vi "eval.vi"(8 "Environment in":T1, 9 "Expression in":T2) -> (2 "Environment out":T1, 3 "Expression out":T2)   [LabVIEW 2020]
uses:
  ExpressionType.ctl
  Expression.ctl
  ClosureData.ctl
  Environment.ctl
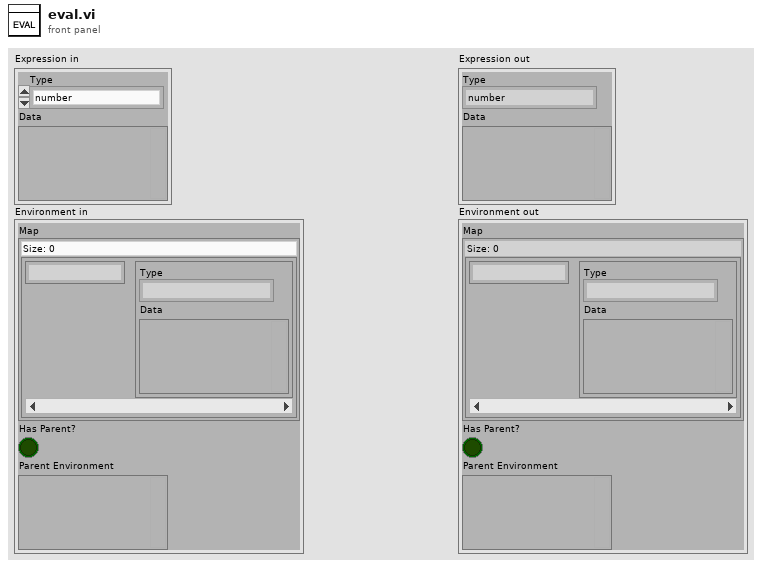
[diagram p1: front panel]
types:
  T1 = typedef "Environment.ctl" = cluster{"Map":map{string, T2}, "Has Parent?":bool, "Parent Environment":variant}
  T2 = typedef "Expression.ctl" = cluster{"Type":T3, "Data":variant}
  T3 = typedef "ExpressionType.ctl" = enum16{"number", "string", "symbol", "primitive", "list", "closure", "macro", "nil", "error"}
  T4 = typedef "ClosureData.ctl" = cluster{"arguments":string[], "code":T2}
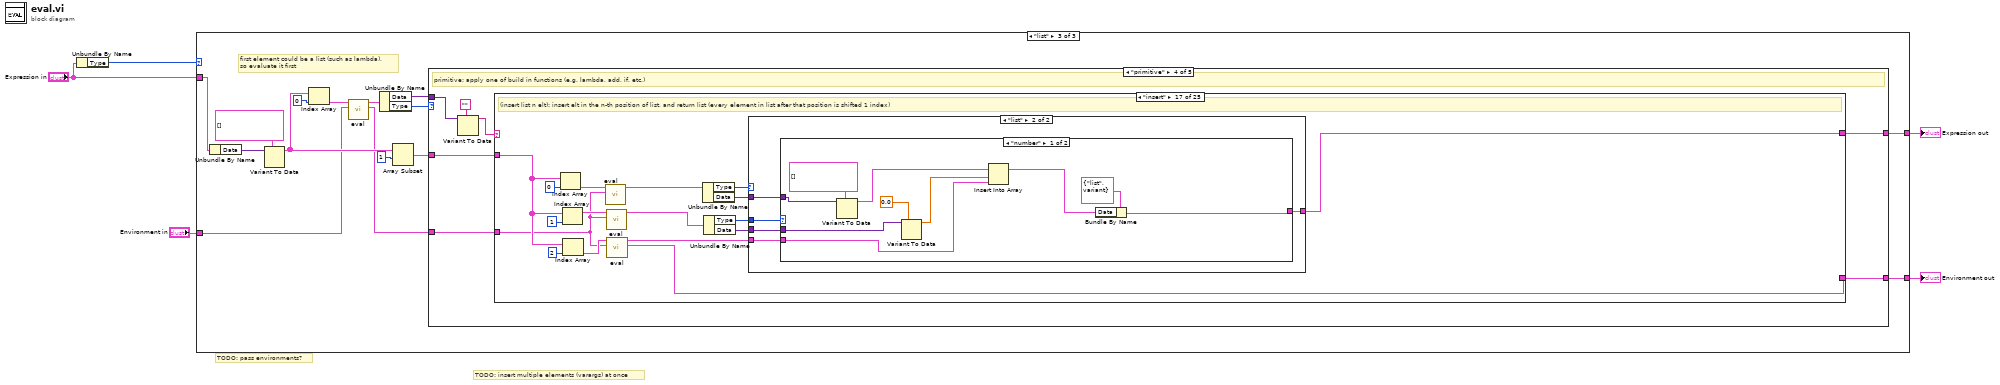
[diagram p0: block diagram]
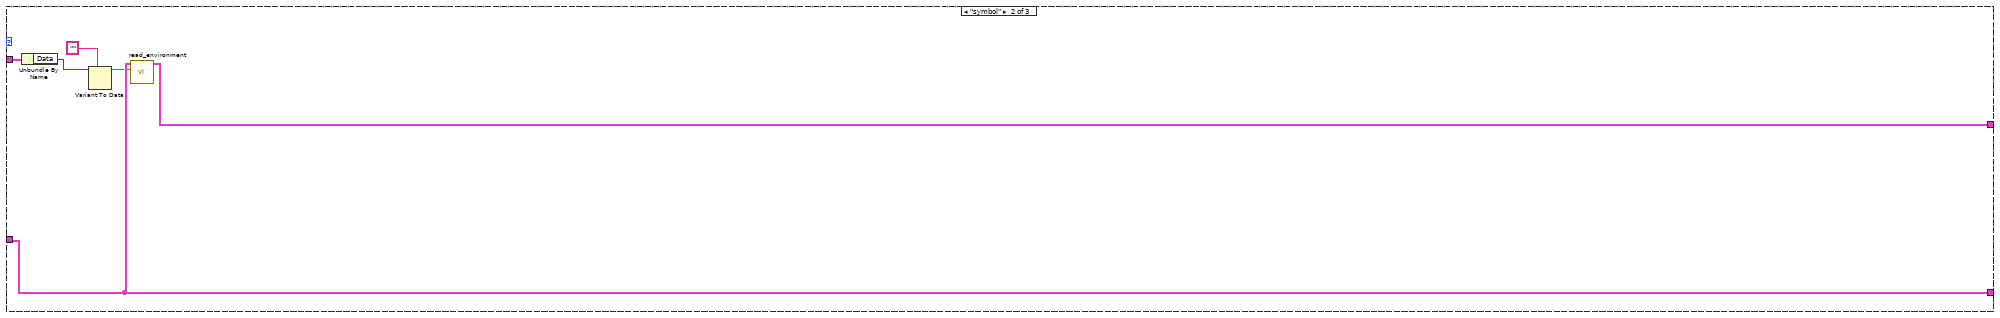
[diagram p3: hidden frame]
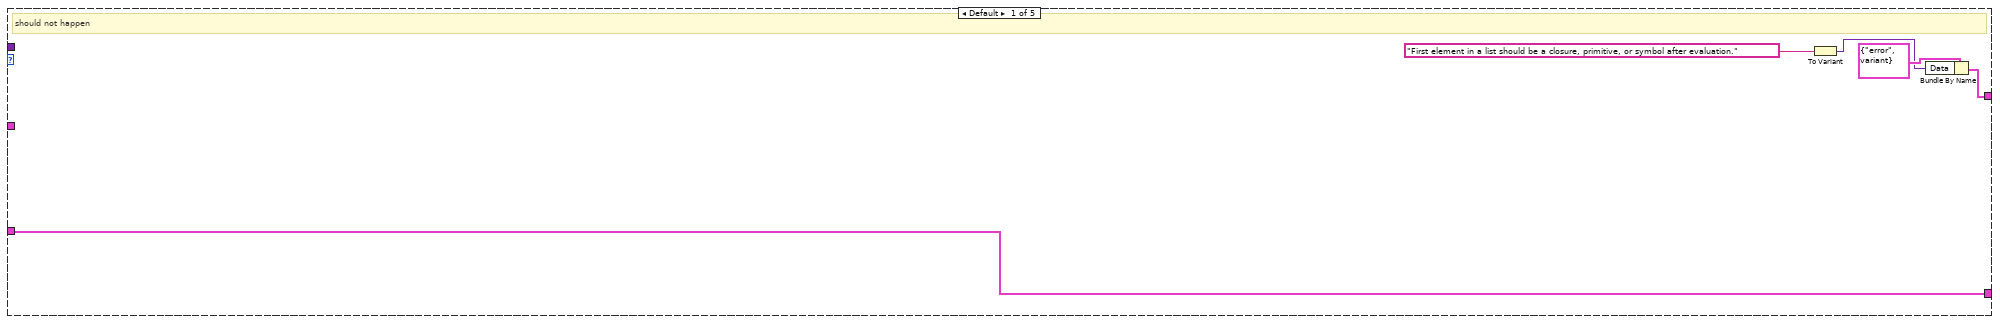
[diagram p4: hidden frame]
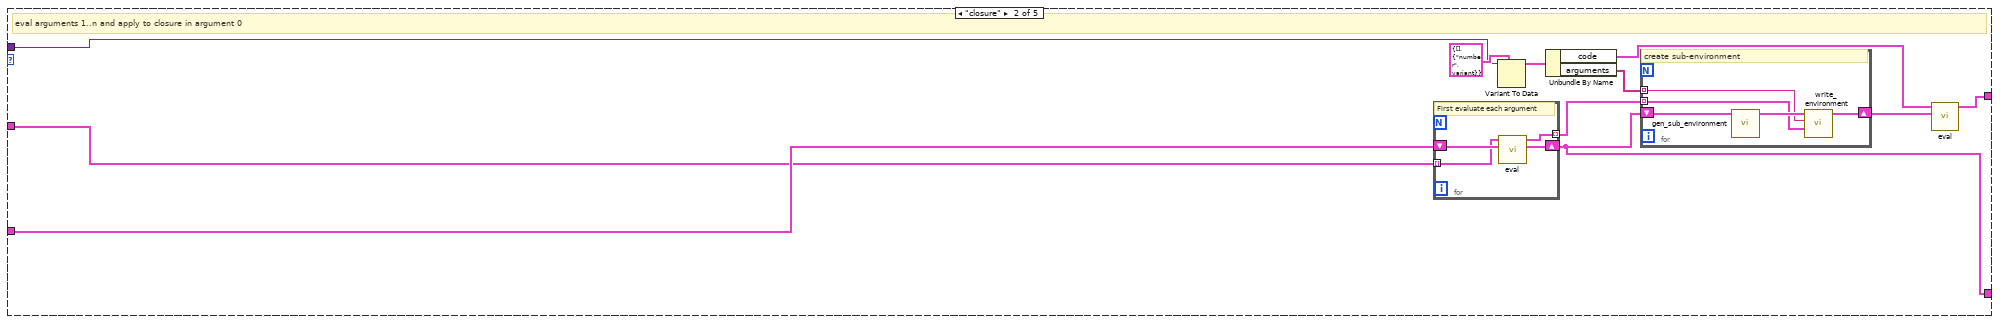
[diagram p5: hidden frame]
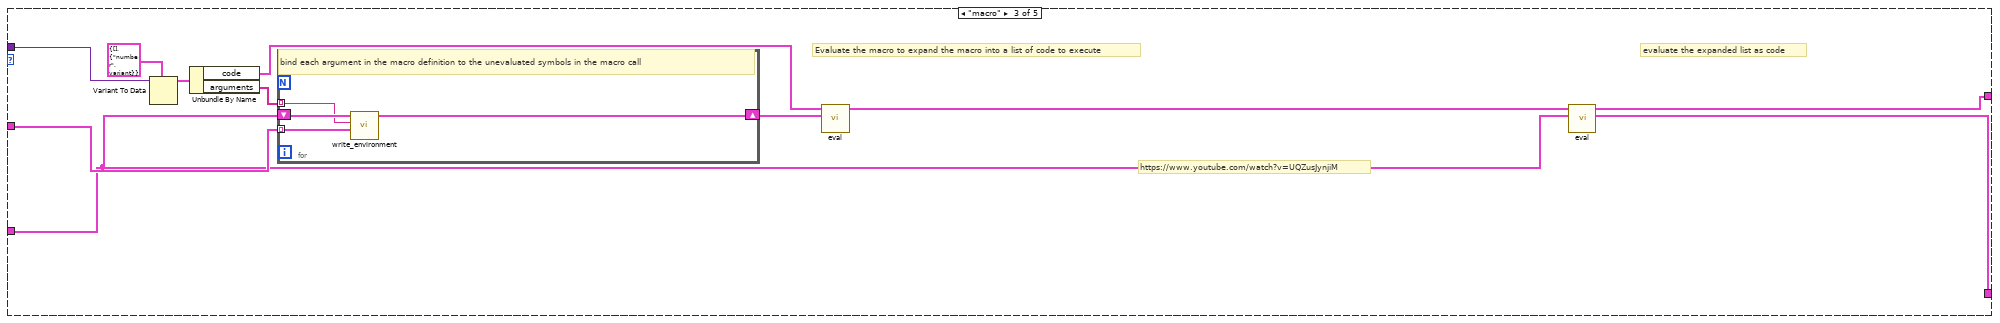
[diagram p6: hidden frame]
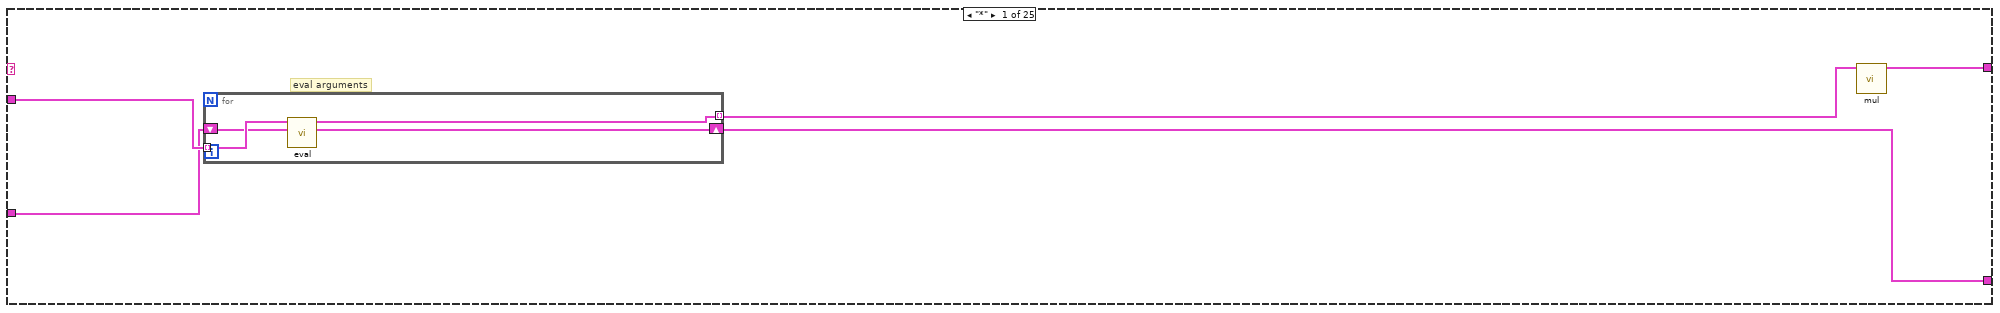
[diagram p7: hidden frame]
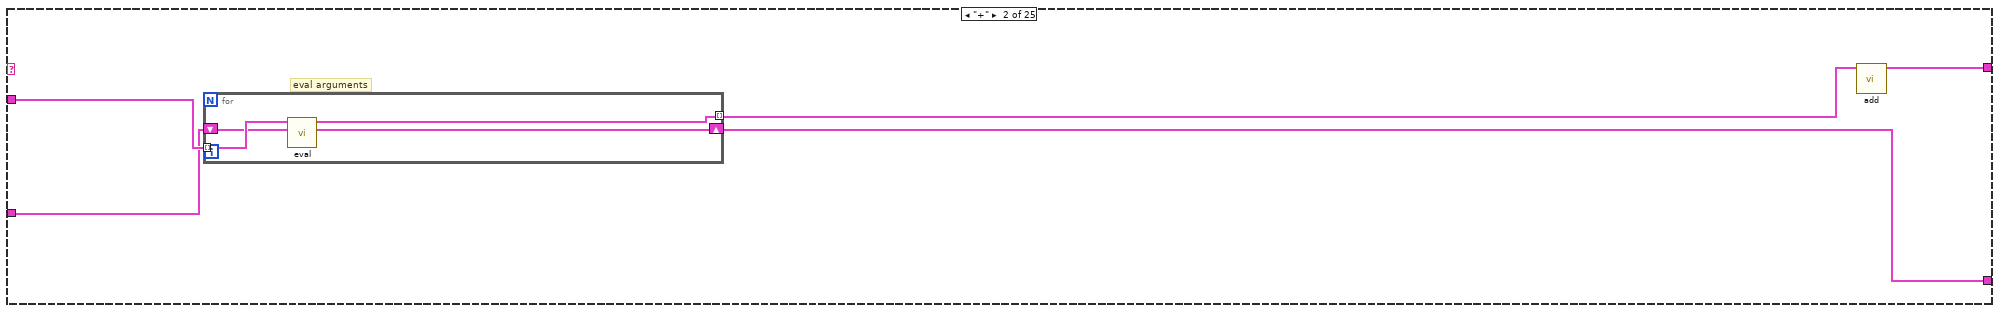
[diagram p8: hidden frame]
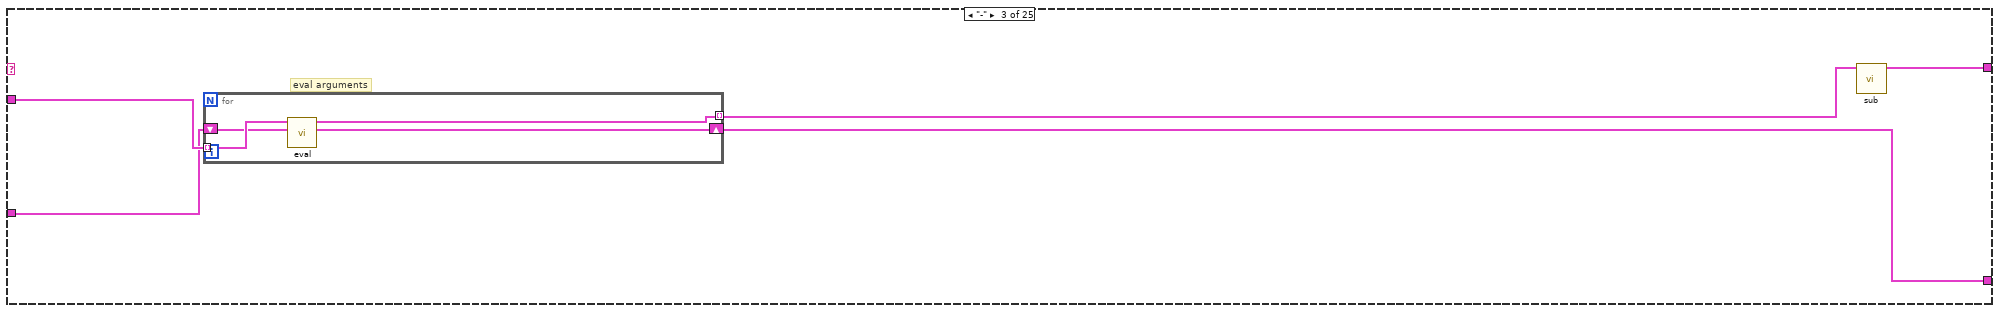
[diagram p9: hidden frame]
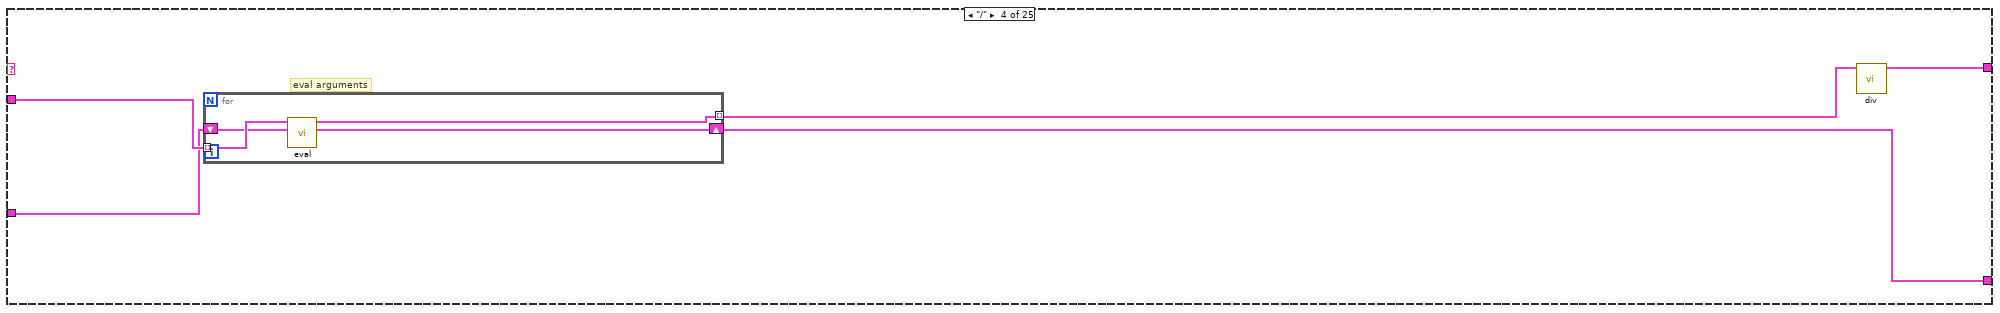
[diagram p10: hidden frame]
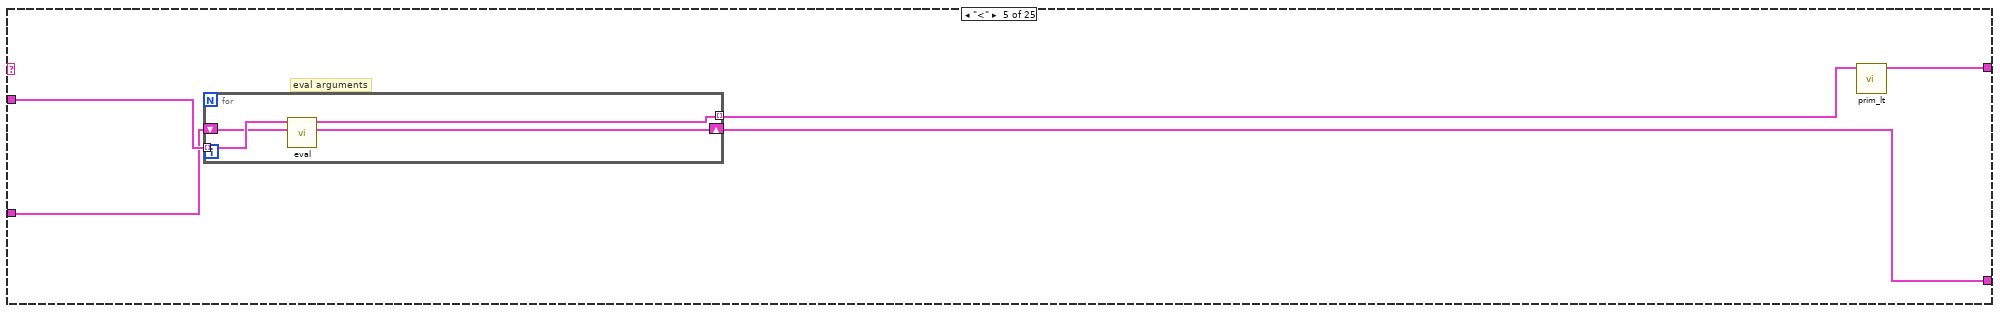
[diagram p11: hidden frame]
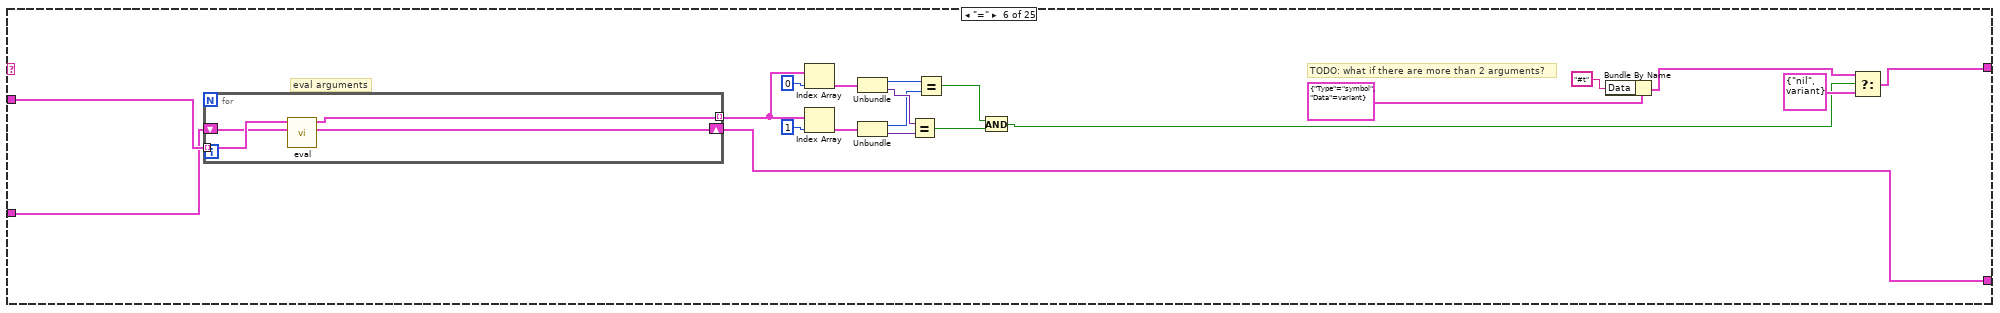
[diagram p12: hidden frame]
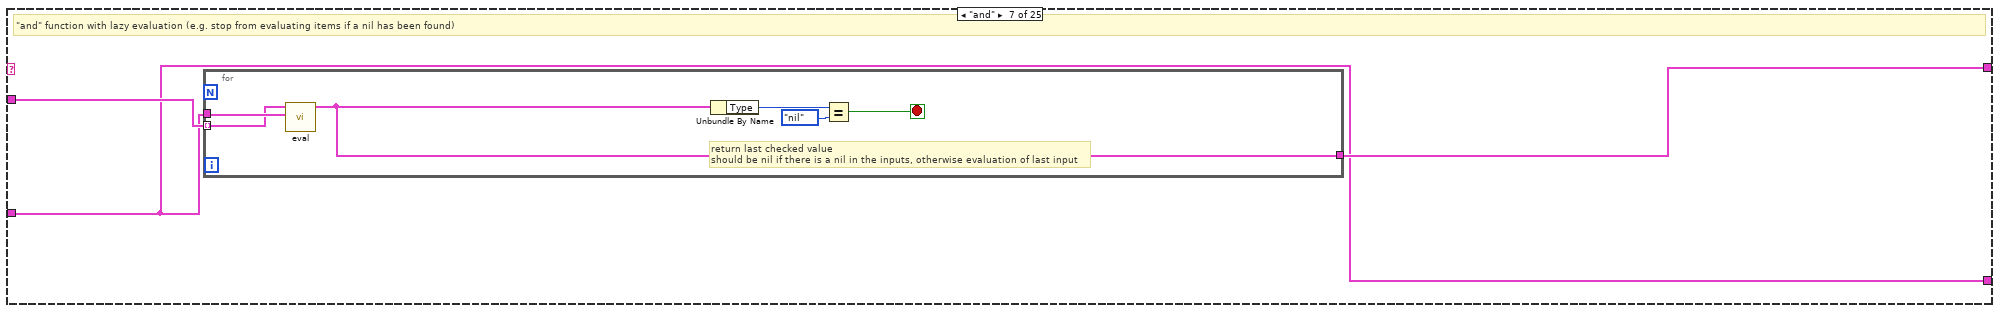
[diagram p13: hidden frame]
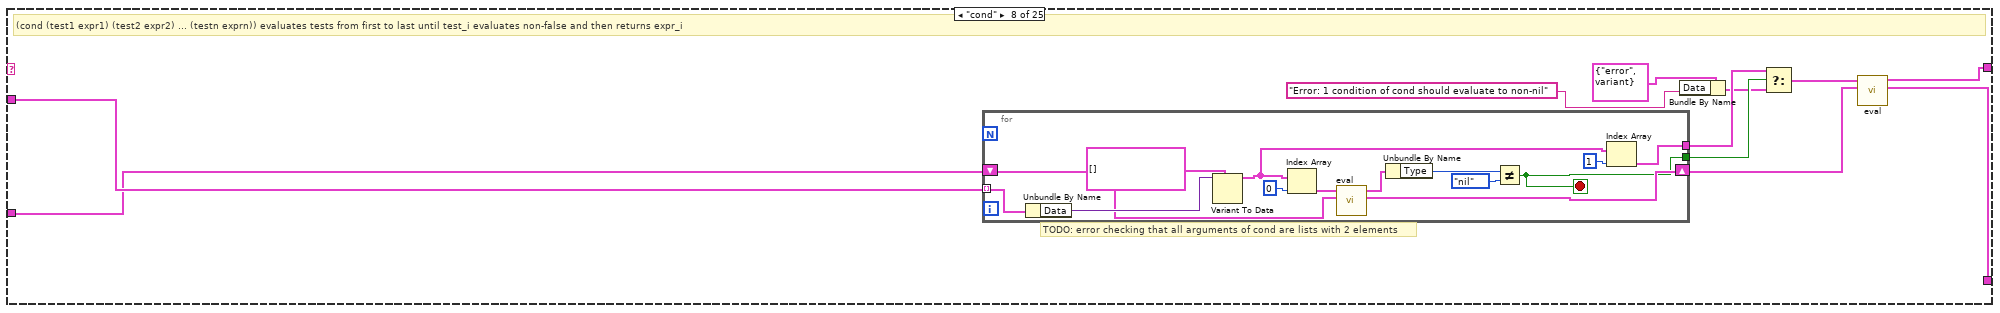
[diagram p14: hidden frame]
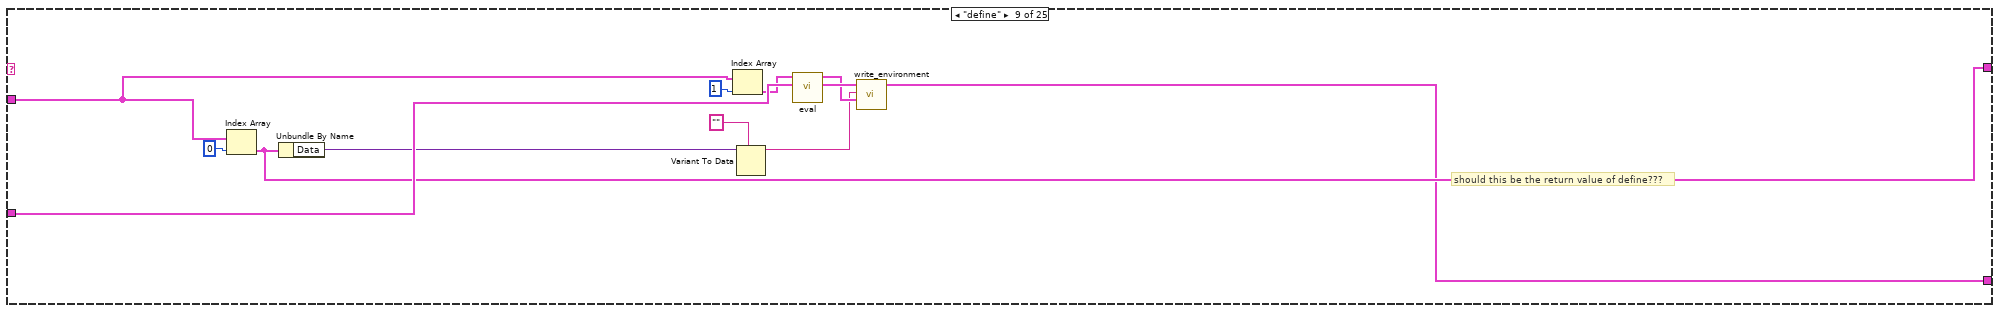
[diagram p15: hidden frame]
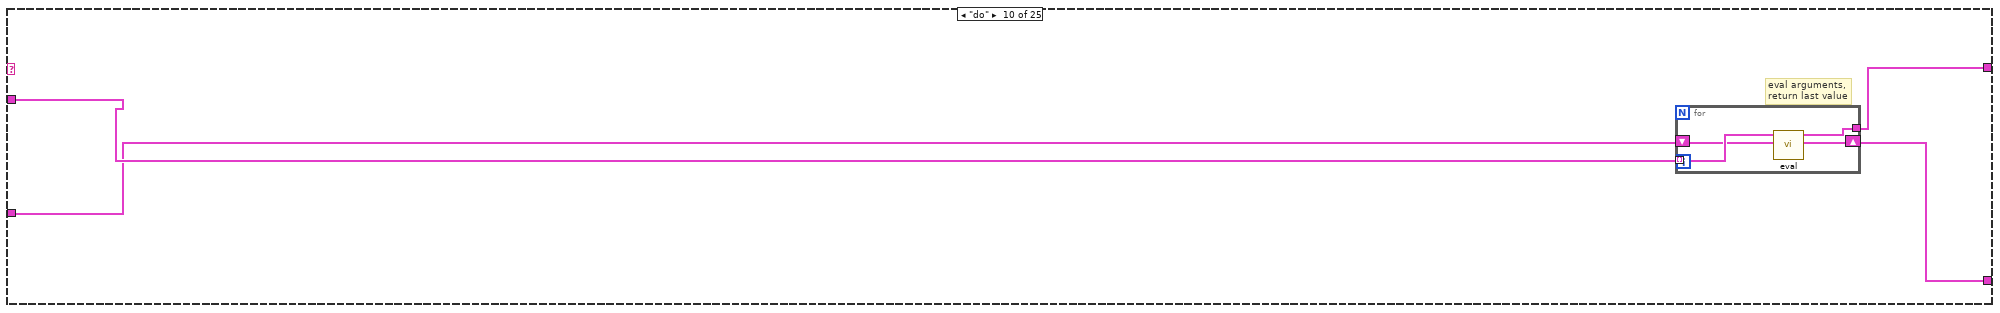
[diagram p16: hidden frame]
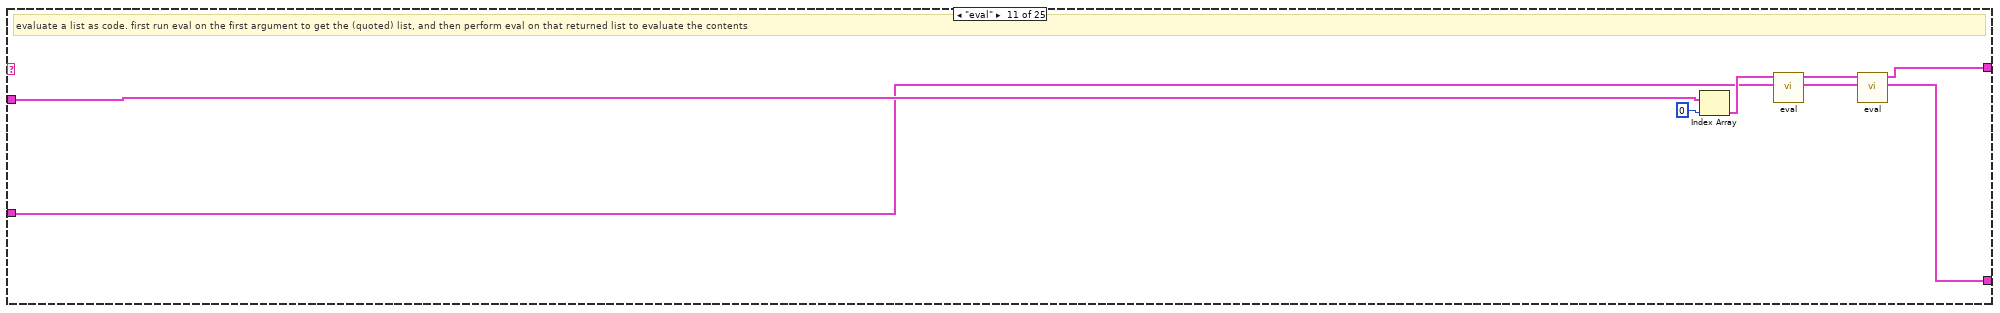
[diagram p17: hidden frame]
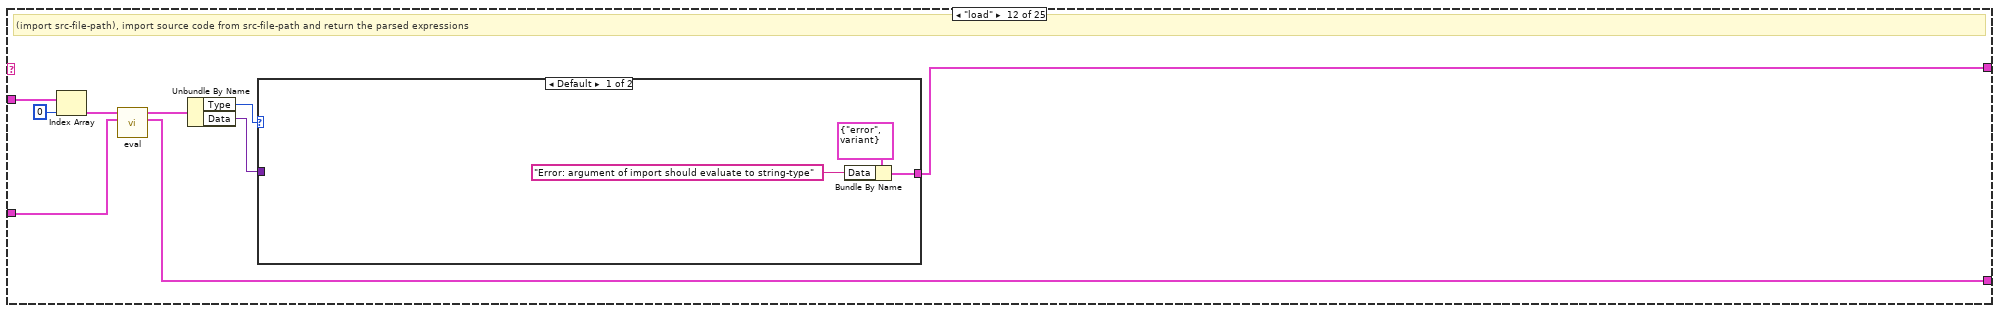
[diagram p18: hidden frame]
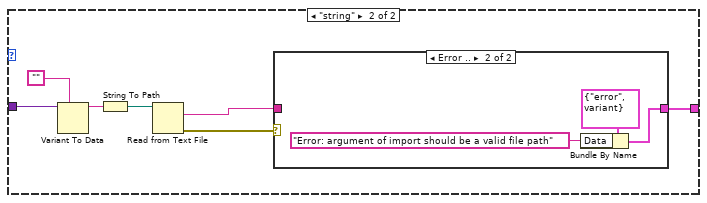
[diagram p19: hidden frame]
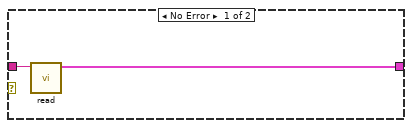
[diagram p20: hidden frame]
diagram:
  # "TODO: insert multiple elements (varargs) at once"
  # "TODO: pass environments?"
  n1 = Unbundle By Name("Expression in") -> ("Type"=w4:T3)
  n2 = case shown="\"list\"" w4 {
    tunnel: "Expression in" -> [w7 w9 w15]
    tunnel: [w7 w11 w25] -> w3
    tunnel: "Environment in" -> [w6 w12 w17]
    tunnel: [w6 w12 w16] -> w1
    frame "number", "string", "primitive", "closure".."error" {
    }
    frame "symbol" {
      n3 = Unbundle By Name(w9) -> ("Data"=w8:variant)
      n4 = Variant To Data(type="", Variant=w8) -> (data=w10:string)  [unwired: 1 in, 1 out]
      n5 = call "read_environment.vi"("symbol"=w10, "Environment in"=w12) -> ("Expression"=w11:T2)  [unwired: 9 in]
    }
    frame "list" {
      # "first element could be a list (such as lambda),\nso evaluate it first"
      n6 = Unbundle By Name(w15) -> ("Data"=w14:variant)
      n7 = Variant To Data(type=T2[] [], Variant=w14) -> (data=w23:T2[])  [unwired: 1 in, 1 out]
      n8 = Index Array(array=w23, index=0) -> (element=w19:T2)
      n9 = call "eval.vi"("Environment in"=w17, "Expression in"=w19) -> ("Environment out"=w20:T1, "Expression out"=w18:T2)  [unwired: 6 in]
      n10 = Unbundle By Name(w18) -> ("Data"=w26:variant, "Type"=w21:T3)
      n11 = Array Subset(array=w23, index=1) -> (w22:T2[])  [unwired: 1 in]
      n12 = case shown="\"primitive\"" w21 {
        tunnel: w26 -> [_ w41 w63 w74 w476]
        tunnel: w20 -> [w33 w44 w57 w70 w474]
        tunnel: [w29 w34 w54 w72 w472] -> w25
        tunnel: w22 -> [_ w43 w60 w71 _]
        tunnel: [w33 w37 w55 w69 w474] -> w16
        frame Default {
          # "should not happen"
          n13 = To Variant(anything="First element in a list should be a closure, primitive, or symbol after evaluation.") -> (Variant=w31:variant)
          n14 = Bundle By Name(cluster=T2 {"Type"=enum."error", "Data"=variant} ("Expression out"), "Data"=w31) -> (w29:T2)
        }
        frame "closure" {
          # "eval arguments 1..n and apply to closure in argument 0"
          n15 = for {
            shift-right: [w52] -> w37
            shift-left: w44 -> [w53]
            tunnel: w43 -> [w51] mode=indexing
            tunnel: [w50] -> w39 mode=indexing
            # "First evaluate each argument"
            n16 = call "eval.vi"("Environment in"=w53, "Expression in"=w51) -> ("Environment out"=w52:T1, "Expression out"=w50:T2)  [unwired: 6 in]
          }
          n17 = Variant To Data(type=T4 {"arguments"=[], "code"={"Type"=enum."number", "Data"=variant}} ("ClosureData"), Variant=w41) -> (data=w40:T4)  [unwired: 1 in, 1 out]
          n18 = Unbundle By Name(w40) -> ("code"=w35:T2, "arguments"=w38:string[])
          n19 = for {
            tunnel: w39 -> [w45] mode=indexing
            tunnel: w38 -> [w46] mode=indexing
            shift-right: [w47] -> w36
            shift-left: w37 -> [w49]
            # "create sub-environment"
            n20 = call "gen_sub_environment.vi"("Environment in"=w49) -> ("Environment out"=w48:T1)  [unwired: 10 in]
            n21 = call "write_environment.vi"("Expression"=w45, "symbol"=w46, "Environment in"=w48) -> ("Environment out"=w47:T1)  [unwired: 8 in]
          }
          n22 = call "eval.vi"("Environment in"=w36, "Expression in"=w35) -> ("Expression out"=w34:T2)  [unwired: 6 in, 1 out]
        }
        frame "macro" {
          # "evaluate the expanded list as code"
          # "Evaluate the macro to expand the macro into a list of code to execute"
          # "https://www.youtube.com/watch?v=UQZusJynjiM"
          n23 = Variant To Data(type=T4 {"arguments"=[], "code"={"Type"=enum."number", "Data"=variant}} ("ClosureData"), Variant=w63) -> (data=w62:T4)  [unwired: 1 in, 1 out]
          n24 = Unbundle By Name(w62) -> ("code"=w59:T2, "arguments"=w61:string[])
          n25 = for {
            tunnel: w61 -> [w66] mode=indexing
            shift-right: [w67] -> w58
            shift-left: w57 -> [w68]
            tunnel: w60 -> [w65] mode=indexing
            # "bind each argument in the macro definition to the unevaluated symbols in the macro call"
            n26 = call "write_environment.vi"("Expression"=w65, "symbol"=w66, "Environment in"=w68) -> ("Environment out"=w67:T1)  [unwired: 8 in]
          }
          n27 = call "eval.vi"("Environment in"=w58, "Expression in"=w59) -> ("Expression out"=w56:T2)  [unwired: 6 in, 1 out]
          n28 = call "eval.vi"("Environment in"=w57, "Expression in"=w56) -> ("Environment out"=w55:T1, "Expression out"=w54:T2)  [unwired: 6 in]
        }
        frame "primitive" {
          # "primitive: apply one of build in functions (e.g. lambda, add, if, etc.)"
          n29 = Variant To Data(type="", Variant=w74) -> (data=w73:string)  [unwired: 1 in, 1 out]
          n30 = case shown="\"insert\"" w73 {
            tunnel: [w80 w89 w98 w107 w116 w121 w146 w158 w183 w191 w199 w207 w242 w252 w275 w293 w328 w362 w381 w419 w427 w435 w441 w447 T2 {"Type"=enum."error", "Data"=variant} ("Expression 3")] -> w72
            tunnel: w71 -> [w79 w88 w97 w106 w115 w140 w147 w164 w186 w194 w205 w214 w235 w257 w280 w289 w320 w358 w377 w412 w428 w439 w442 w445 _]
            tunnel: w70 -> [w78 w87 w96 w105 w114 w139 w145 w163 w190 w193 w203 w213 w240 w251 w279 w292 w318 w361 w380 w417 w426 w437 w444 w449 w470]
            tunnel: [w76 w85 w94 w103 w112 w138 w145 w159 w182 w192 w200 w212 w240 w251 w276 w298 w317 w354 w386 w417 w426 w436 w444 w448 w470] -> w69
            frame "*" {
              # "eval arguments"
              n31 = for {
                tunnel: w79 -> [w84] mode=indexing
                tunnel: [w82] -> w77 mode=indexing
                shift-right: [w81] -> w76
                shift-left: w78 -> [w83]
                n32 = call "eval.vi"("Environment in"=w83, "Expression in"=w84) -> ("Environment out"=w81:T1, "Expression out"=w82:T2)  [unwired: 6 in]
              }
              n33 = call "mul.vi"("arguments"=w77) -> ("Expression"=w80:T2)  [unwired: 10 in]
            }
            frame "+" {
              # "eval arguments"
              n34 = for {
                tunnel: w88 -> [w93] mode=indexing
                tunnel: [w91] -> w86 mode=indexing
                shift-right: [w90] -> w85
                shift-left: w87 -> [w92]
                n35 = call "eval.vi"("Environment in"=w92, "Expression in"=w93) -> ("Environment out"=w90:T1, "Expression out"=w91:T2)  [unwired: 6 in]
              }
              n36 = call "add.vi"("arguments"=w86) -> ("Expression"=w89:T2)  [unwired: 10 in]
            }
            frame "-" {
              # "eval arguments"
              n37 = for {
                tunnel: w97 -> [w102] mode=indexing
                tunnel: [w100] -> w95 mode=indexing
                shift-right: [w99] -> w94
                shift-left: w96 -> [w101]
                n38 = call "eval.vi"("Environment in"=w101, "Expression in"=w102) -> ("Environment out"=w99:T1, "Expression out"=w100:T2)  [unwired: 6 in]
              }
              n39 = call "sub.vi"("arguments"=w95) -> ("Expression"=w98:T2)  [unwired: 10 in]
            }
            frame "/" {
              # "eval arguments"
              n40 = for {
                tunnel: w106 -> [w111] mode=indexing
                tunnel: [w109] -> w104 mode=indexing
                shift-right: [w108] -> w103
                shift-left: w105 -> [w110]
                n41 = call "eval.vi"("Environment in"=w110, "Expression in"=w111) -> ("Environment out"=w108:T1, "Expression out"=w109:T2)  [unwired: 6 in]
              }
              n42 = call "div.vi"("arguments"=w104) -> ("Expression"=w107:T2)  [unwired: 10 in]
            }
            frame "<" {
              # "eval arguments"
              n43 = for {
                tunnel: w115 -> [w120] mode=indexing
                tunnel: [w118] -> w113 mode=indexing
                shift-right: [w117] -> w112
                shift-left: w114 -> [w119]
                n44 = call "eval.vi"("Environment in"=w119, "Expression in"=w120) -> ("Environment out"=w117:T1, "Expression out"=w118:T2)  [unwired: 6 in]
              }
              n45 = call "prim_lt.vi"("arguments"=w113) -> ("Expression out"=w116:T2)  [unwired: 10 in]
            }
            frame "=" {
              # "TODO: what if there are more than 2 arguments?"
              # "eval arguments"
              n46 = for {
                tunnel: w140 -> [w144] mode=indexing
                tunnel: [w142] -> w133 mode=indexing
                shift-right: [w141] -> w138
                shift-left: w139 -> [w143]
                n47 = call "eval.vi"("Environment in"=w143, "Expression in"=w144) -> ("Environment out"=w141:T1, "Expression out"=w142:T2)  [unwired: 6 in]
              }
              n48 = Index Array(array=w133, index=0) -> (element=w130:T2)
              n49 = Index Array(array=w133, index=1) -> (element=w129:T2)
              n50 = Unbundle(w130) -> ("Type"=w128:T3, "Data"=w126:variant)
              n51 = Unbundle(w129) -> ("Type"=w125:T3, "Data"=w127:variant)
              n52 = Equal?(x=w126, y=w127) -> (x = y?=w123:bool)
              n53 = Equal?(x=w128, y=w125) -> (x = y?=w124:bool)
              n54 = And(x=w124, y=w123) -> (x .and. y?=w122:bool)
              n55 = Bundle By Name(cluster=T2 {"Type"=enum."symbol", "Data"=variant} ("Expression 3"), "Data"="#t") -> (w137:T2)
              n56 = Select(t=w137, s=w122, f=T2 {"Type"=enum."nil", "Data"=variant} ("Expression 3")) -> (s? t:f=w121:T2)
            }
            frame "and" {
              # "\"and\" function with lazy evaluation (e.g. stop from evaluating items if a nil has been found)"
              n57 = for {
                tunnel: w145 -> [w151]
                tunnel: w147 -> [w150] mode=indexing
                tunnel: [w148] -> w146
                stop <- w149 stop-if-true
                # "return last checked value\nshould be nil if there is a nil in the inputs, otherwise evaluation of last input"
                n58 = call "eval.vi"("Environment in"=w151, "Expression in"=w150) -> ("Expression out"=w148:T2)  [unwired: 6 in, 1 out]
                n59 = Unbundle By Name(w148) -> ("Type"=w153:T3)
                n60 = Equal?(x=w153, y=ExpressionType."nil") -> (x = y?=w149:bool)
              }
            }
            frame "cond" {
              # "TODO: error checking that all arguments of cond are lists with 2 elements"
              # "(cond (test1 expr1) (test2 expr2) ... (testn exprn)) evaluates tests from first to last until test_i evaluates non-false and then returns expr_i"
              n61 = for {
                tunnel: w164 -> [w177] mode=indexing
                shift-right: [w170] -> w155
                shift-left: w163 -> [w169]
                tunnel: [w166] -> w162
                tunnel: [w165] -> w161
                stop <- w166 stop-if-true
                n62 = Unbundle By Name(w177) -> ("Data"=w176:variant)
                n63 = Variant To Data(type=T2[] [], Variant=w176) -> (data=w173:T2[])  [unwired: 1 in, 1 out]
                n64 = Index Array(array=w173, index=0) -> (element=w172:T2)
                n65 = call "eval.vi"("Environment in"=w169, "Expression in"=w172) -> ("Environment out"=w170:T1, "Expression out"=w171:T2)  [unwired: 6 in]
                n66 = Unbundle By Name(w171) -> ("Type"=w168:T3)
                n67 = Not Equal?(x=w168, y=ExpressionType."nil") -> (x != y?=w166:bool)
                n68 = Index Array(array=w173, index=1) -> (element=w165:T2)
              }
              n69 = Bundle By Name(cluster=T2 {"Type"=enum."error", "Data"=variant} ("Expression in"), "Data"="Error: 1 condition of cond should evaluate to non-nil") -> (w157:T2)
              n70 = Select(t=w161, s=w162, f=w157) -> (s? t:f=w160:T2)
              n71 = call "eval.vi"("Environment in"=w155, "Expression in"=w160) -> ("Environment out"=w159:T1, "Expression out"=w158:T2)  [unwired: 6 in]
            }
            frame "define" {
              # "should this be the return value of define???"
              n72 = Index Array(array=w186, index=0) -> (element=w183:T2)
              n73 = Unbundle By Name(w183) -> ("Data"=w185:variant)
              n74 = Index Array(array=w186, index=1) -> (element=w188:T2)
              n75 = Variant To Data(type="", Variant=w185) -> (data=w179:string)  [unwired: 1 in, 1 out]
              n76 = call "eval.vi"("Environment in"=w190, "Expression in"=w188) -> ("Environment out"=w181:T1, "Expression out"=w180:T2)  [unwired: 6 in]
              n77 = call "write_environment.vi"("Expression"=w180, "symbol"=w179, "Environment in"=w181) -> ("Environment out"=w182:T1)  [unwired: 8 in]
            }
            frame "do" {
              # "eval arguments,\nreturn last value"
              n78 = for {
                tunnel: w194 -> [w198] mode=indexing
                tunnel: [w196] -> w191
                shift-right: [w195] -> w192
                shift-left: w193 -> [w197]
                n79 = call "eval.vi"("Environment in"=w197, "Expression in"=w198) -> ("Environment out"=w195:T1, "Expression out"=w196:T2)  [unwired: 6 in]
              }
            }
            frame "eval" {
              # "evaluate a list as code. first run eval on the first argument to get the (quoted) list, and then perform eval on that returned list to evaluate the contents"
              n80 = Index Array(array=w205, index=0) -> (element=w204:T2)
              n81 = call "eval.vi"("Environment in"=w203, "Expression in"=w204) -> ("Environment out"=w202:T1, "Expression out"=w201:T2)  [unwired: 6 in]
              n82 = call "eval.vi"("Environment in"=w202, "Expression in"=w201) -> ("Environment out"=w200:T1, "Expression out"=w199:T2)  [unwired: 6 in]
            }
            frame "load" {
              # "(import src-file-path), import source code from src-file-path and return the parsed expressions"
              n83 = Index Array(array=w214, index=0) -> (element=w215:T2)
              n84 = call "eval.vi"("Environment in"=w213, "Expression in"=w215) -> ("Environment out"=w212:T1, "Expression out"=w210:T2)  [unwired: 6 in]
              n85 = Unbundle By Name(w210) -> ("Type"=w209:T3, "Data"=w208:variant)
              n86 = case shown="Default" w209 {
                tunnel: w208 -> [_ w225]
                tunnel: [w216 w221] -> w207
                frame Default {
                  n87 = Bundle By Name(cluster=T2 {"Type"=enum."error", "Data"=variant} ("Expression in"), "Data"="Error: argument of import should evaluate to string-type") -> (w216:T2)
                }
                frame "string" {
                  n88 = Variant To Data(type="", Variant=w225) -> (data=w220:string)  [unwired: 1 in, 1 out]
                  n89 = String To Path(string=w220) -> (path=w219:path)
                  n90 = Read from Text File(file (use dialog)=w219) -> (text=w222:string, error out=w223:errorcluster)  [unwired: 3 in, 2 out]
                  n91 = case shown="Error .." w223 {
                    tunnel: w222 -> [w227 _]
                    tunnel: [w226 w228] -> w221
                    frame No Error {
                      n92 = call "read.vi"("input string"=w227) -> ("Expression out"=w226:T2)  [unwired: 10 in]
                    }
                    frame Error {
                      n93 = Bundle By Name(cluster=T2 {"Type"=enum."error", "Data"=variant} ("Expression in"), "Data"="Error: argument of import should be a valid file path") -> (w228:T2)
                    }
                  }
                }
              }
            }
            frame "lambda" {
              # "extract names from list of symbols"
              n94 = Index Array(array=w235, index=0) -> (element=w234:T2)
              n95 = Unbundle By Name(w234) -> ("Data"=w232:variant)
              n96 = Variant To Data(type=T2[] [], Variant=w232) -> (data=w231:T2[])  [unwired: 1 in, 1 out]
              n97 = for {
                tunnel: w231 -> [w248] mode=indexing
                tunnel: [w245] -> w239 mode=indexing
                n98 = Unbundle By Name(w248) -> ("Data"=w247:variant)
                n99 = Variant To Data(type="", Variant=w247) -> (data=w245:string)  [unwired: 1 in, 1 out]
              }
              n100 = Index Array(array=w235, index=1) -> (element=w237:T2)
              n101 = Bundle By Name(cluster=T4 {"arguments"=[], "code"={"Type"=enum."number", "Data"=variant}} ("ClosureData"), "arguments"=w239, "code"=w237) -> (w241:T4)
              n102 = Bundle By Name(cluster=T2 {"Type"=enum."closure", "Data"=variant} ("Expression 3"), "Data"=w241) -> (w242:T2)
            }
            frame "let" {
              # "expr"
              # "list of var definitions"
              # "(let ((var1 expr1) (var2 expr2) .. (varn exprn)) expr) defines local variables (in order) var_x for use in scope of expr"
              n103 = Index Array(array=w257, index=0) -> (element=w256:T2)
              n104 = Unbundle By Name(w256) -> ("Data"=w254:variant)
              n105 = Variant To Data(type=T2[] [], Variant=w254) -> (data=w253:T2[])  [unwired: 1 in, 1 out]
              n106 = for {
                tunnel: w253 -> [w262] mode=indexing
                shift-right: [w265] -> w250
                shift-left: w251 -> [w260]
                # "var definition"
                # "evaluate expr_x and add to env"
                n107 = Unbundle By Name(w262) -> ("Data"=w263:variant)
                n108 = Variant To Data(type=T2[] [], Variant=w263) -> (data=w261:T2[])  [unwired: 1 in, 1 out]
                n109 = Index Array(array=w261, index=0) -> (element=w271:T2)
                n110 = Unbundle By Name(w271) -> ("Data"=w270:variant)
                n111 = Index Array(array=w261, index=1) -> (element=w269:T2)
                n112 = Variant To Data(type="", Variant=w270) -> (data=w274:string)  [unwired: 1 in, 1 out]
                n113 = call "eval.vi"("Environment in"=w260, "Expression in"=w269) -> ("Environment out"=w272:T1, "Expression out"=w273:T2)  [unwired: 6 in]
                n114 = call "write_environment.vi"("Expression"=w273, "symbol"=w274, "Environment in"=w272) -> ("Environment out"=w265:T1)  [unwired: 8 in]
              }
              n115 = Index Array(array=w257, index=1) -> (element=w249:T2)
              n116 = call "eval.vi"("Environment in"=w250, "Expression in"=w249) -> ("Expression out"=w252:T2)  [unwired: 6 in, 1 out]
            }
            frame "list" {
              # "eval arguments,\nreturn last value"
              # "Create new list with evaluated objects"
              n117 = for {
                tunnel: w280 -> [w284] mode=indexing
                tunnel: [w282] -> w277 mode=indexing
                shift-right: [w281] -> w276
                shift-left: w279 -> [w283]
                n118 = call "eval.vi"("Environment in"=w283, "Expression in"=w284) -> ("Environment out"=w281:T1, "Expression out"=w282:T2)  [unwired: 6 in]
              }
              n119 = Bundle By Name(cluster=T2 {"Type"=enum."list", "Data"=variant} ("Expression out"), "Data"=w277) -> (w275:T2)
            }
            frame "nth" {
              # "(nth n list): return list[n]"
              n120 = Index Array(array=w289, index=0) -> (element=w290:T2)
              n121 = Index Array(array=w289, index=1) -> (element=w295:T2)
              n122 = call "eval.vi"("Environment in"=w292, "Expression in"=w290) -> ("Expression out"=w287:T2)  [unwired: 6 in, 1 out]
              n123 = call "eval.vi"("Environment in"=w292, "Expression in"=w295) -> ("Environment out"=w298:T1, "Expression out"=w294:T2)  [unwired: 6 in]
              n124 = Unbundle By Name(w287) -> ("Type"=w288:T3, "Data"=w286:variant)
              n125 = Unbundle By Name(w294) -> ("Type"=w297:T3, "Data"=w285:variant)
              n126 = case shown="\"number\"" w288 {
                tunnel: w297 -> [_ w305]
                tunnel: [w299 w304] -> w293
                tunnel: w286 -> [_ w303]
                tunnel: w285 -> [_ w302]
                frame Default {
                  n127 = Bundle By Name(cluster=T2 {"Type"=enum."error", "Data"=variant} ("Expression in"), "Data"="Error: first argument of nth should be number-type") -> (w299:T2)
                }
                frame "number" {
                  n128 = case shown="Default" w305 {
                    tunnel: [w306 w313] -> w304
                    tunnel: w303 -> [w311 _]
                    tunnel: w302 -> [w309 _]
                    frame "list" {
                      n129 = Variant To Data(type=0.0, Variant=w311) -> (data=w310:dbl)  [unwired: 1 in, 1 out]
                      n130 = Variant To Data(type=T2[] [], Variant=w309) -> (data=w307:T2[])  [unwired: 1 in, 1 out]
                      n131 = Index Array(array=w307, index=w310) -> (element=w306:T2)
                    }
                    frame Default {
                      n132 = Bundle By Name(cluster=T2 {"Type"=enum."error", "Data"=variant} ("Expression in"), "Data"="Error: second argument of nth should be list-type") -> (w313:T2)
                    }
                  }
                }
              }
            }
            frame "insert" {
              # "(insert list n elt): insert elt in the n-th position of list, and return list (every element in list after that position is shifted 1 index)"
              n133 = Index Array(array=w320, index=0) -> (element=w326:T2)
              n134 = Index Array(array=w320, index=1) -> (element=w330:T2)
              n135 = Index Array(array=w320, index=2) -> (element=w319:T2)
              n136 = call "eval.vi"("Environment in"=w318, "Expression in"=w326) -> ("Expression out"=w324:T2)  [unwired: 6 in, 1 out]
              n137 = call "eval.vi"("Environment in"=w318, "Expression in"=w330) -> ("Expression out"=w329:T2)  [unwired: 6 in, 1 out]
              n138 = call "eval.vi"("Environment in"=w318, "Expression in"=w319) -> ("Environment out"=w317:T1, "Expression out"=w316:T2)  [unwired: 6 in]
              n139 = Unbundle By Name(w324) -> ("Type"=w325:T3, "Data"=w323:variant)
              n140 = Unbundle By Name(w329) -> ("Type"=w332:T3, "Data"=w322:variant)
              n141 = case shown="\"list\"" w325 {
                tunnel: w332 -> [_ w340]
                tunnel: [w333 w339] -> w328
                tunnel: w323 -> [_ w338]
                tunnel: w322 -> [_ w337]
                tunnel: w316 -> [_ w336]
                frame Default {
                  n142 = Bundle By Name(cluster=T2 {"Type"=enum."error", "Data"=variant} ("Expression in"), "Data"="Error: first argument of insert should be list-type") -> (w333:T2)
                }
                frame "list" {
                  n143 = case shown="\"number\"" w340 {
                    tunnel: [w343 w351] -> w339
                    tunnel: w338 -> [w342 _]
                    tunnel: w337 -> [w341 _]
                    tunnel: w336 -> [w346 _]
                    frame "number" {
                      n144 = Variant To Data(type=T2[] [], Variant=w342) -> (data=w348:T2[])  [unwired: 1 in, 1 out]
                      n145 = Variant To Data(type=0.0, Variant=w341) -> (data=w347:dbl)  [unwired: 1 in, 1 out]
                      n146 = Insert Into Array(array=w348, index=w347, new element=w346) -> (w344:T2[])
                      n147 = Bundle By Name(cluster=T2 {"Type"=enum."list", "Data"=variant} ("Expression out"), "Data"=w344) -> (w343:T2)
                    }
                    frame Default {
                      n148 = Bundle By Name(cluster=T2 {"Type"=enum."error", "Data"=variant} ("Expression in"), "Data"="Error: seconnd argument of insert should be number-type") -> (w351:T2)
                    }
                  }
                }
              }
            }
            frame "len" {
              # "(len list): return length of list"
              n149 = Index Array(array=w358, index=0) -> (element=w359:T2)
              n150 = call "eval.vi"("Environment in"=w361, "Expression in"=w359) -> ("Environment out"=w354:T1, "Expression out"=w356:T2)  [unwired: 6 in]
              n151 = Unbundle By Name(w356) -> ("Type"=w357:T3, "Data"=w355:variant)
              n152 = case shown="\"list\"" w357 {
                tunnel: [w363 w366] -> w362
                tunnel: w355 -> [_ w371]
                frame Default {
                  n153 = Bundle By Name(cluster=T2 {"Type"=enum."error", "Data"=variant} ("Expression in"), "Data"="Error: first argument of len should be list-type") -> (w363:T2)
                }
                frame "list" {
                  n154 = Variant To Data(type=T2[] [], Variant=w371) -> (data=w370:T2[])  [unwired: 1 in, 1 out]
                  n155 = Array Size(array=w370) -> (size(s)=w368:i32)
                  n156 = To Double Precision Float(number=w368) -> (double precision float=w367:dbl)
                  n157 = Bundle By Name(cluster=T2 {"Type"=enum."number", "Data"=variant} ("Expression in"), "Data"=w367) -> (w366:T2)
                }
              }
            }
            frame "nthrest" {
              # "(nthrest n list): return list[n+1:end]"
              n158 = Index Array(array=w377, index=0) -> (element=w378:T2)
              n159 = Index Array(array=w377, index=1) -> (element=w383:T2)
              n160 = call "eval.vi"("Environment in"=w380, "Expression in"=w378) -> ("Expression out"=w375:T2)  [unwired: 6 in, 1 out]
              n161 = call "eval.vi"("Environment in"=w380, "Expression in"=w383) -> ("Environment out"=w386:T1, "Expression out"=w382:T2)  [unwired: 6 in]
              n162 = Unbundle By Name(w375) -> ("Type"=w376:T3, "Data"=w374:variant)
              n163 = Unbundle By Name(w382) -> ("Type"=w385:T3, "Data"=w373:variant)
              n164 = case shown="\"number\"" w376 {
                tunnel: w385 -> [_ w393]
                tunnel: [w387 w392] -> w381
                tunnel: w374 -> [_ w391]
                tunnel: w373 -> [_ w390]
                frame Default {
                  n165 = Bundle By Name(cluster=T2 {"Type"=enum."error", "Data"=variant} ("Expression in"), "Data"="Error: first argument of nthrest should be number-type") -> (w387:T2)
                }
                frame "number" {
                  n166 = case shown="\"list\"" w393 {
                    tunnel: [w397 w405] -> w392
                    tunnel: w391 -> [w403 _]
                    tunnel: w390 -> [w402 _]
                    frame "list" {
                      n167 = Variant To Data(type=0.0, Variant=w403) -> (data=w400:dbl)  [unwired: 1 in, 1 out]
                      n168 = Increment(x=w400) -> (x+1=w394:dbl)
                      n169 = Variant To Data(type=T2[] [], Variant=w402) -> (data=w395:T2[])  [unwired: 1 in, 1 out]
                      n170 = Array Size(array=w395) -> (size(s)=w396:i32)
                      n171 = Array Subset(array=w395, index=w394, length=w396) -> (w398:T2[])
                      n172 = Bundle By Name(cluster=T2 {"Type"=enum."list", "Data"=variant} ("Expression out"), "Data"=w398) -> (w397:T2)
                    }
                    frame Default {
                      n173 = Bundle By Name(cluster=T2 {"Type"=enum."error", "Data"=variant} ("Expression in"), "Data"="Error: second argument of nthrest should be list-type") -> (w405:T2)
                    }
                  }
                }
              }
            }
            frame "macro" {
              # "extract names from list of symbols"
              n174 = Index Array(array=w412, index=0) -> (element=w411:T2)
              n175 = Unbundle By Name(w411) -> ("Data"=w409:variant)
              n176 = Variant To Data(type=T2[] [], Variant=w409) -> (data=w408:T2[])  [unwired: 1 in, 1 out]
              n177 = for {
                tunnel: w408 -> [w425] mode=indexing
                tunnel: [w422] -> w416 mode=indexing
                n178 = Unbundle By Name(w425) -> ("Data"=w424:variant)
                n179 = Variant To Data(type="", Variant=w424) -> (data=w422:string)  [unwired: 1 in, 1 out]
              }
              n180 = Index Array(array=w412, index=1) -> (element=w414:T2)
              n181 = Bundle By Name(cluster=T4 {"arguments"=[], "code"={"Type"=enum."number", "Data"=variant}} ("ClosureData"), "arguments"=w416, "code"=w414) -> (w418:T4)
              n182 = Bundle By Name(cluster=T2 {"Type"=enum."macro", "Data"=variant} ("Expression 3"), "Data"=w418) -> (w419:T2)
            }
            frame "or" {
              # "\"or\" function with lazy evaluation (e.g. stop from evaluating items in a non-nil has been found)"
              n183 = for {
                tunnel: w426 -> [w432]
                tunnel: w428 -> [w431] mode=indexing
                tunnel: [w429] -> w427
                stop <- w430 stop-if-true
                # "return last checked value\nshould be first non-false value, otherwise nil"
                n184 = call "eval.vi"("Environment in"=w432, "Expression in"=w431) -> ("Expression out"=w429:T2)  [unwired: 6 in, 1 out]
                n185 = Unbundle By Name(w429) -> ("Type"=w434:T3)
                n186 = Not Equal?(x=w434, y=ExpressionType."nil") -> (x != y?=w430:bool)
              }
            }
            frame "quasiquote" {
              # "1st (and only) argument is a list. A list with every item is returned, except for the items in form of (unquote var) or (splice-unqote var), which are evaluated"
              n187 = Index Array(array=w439, index=0) -> (element=w438:T2)
              n188 = call "quasiquote_eval.vi"("Environment in"=w437, "Expression in"=w438) -> ("Environment out"=w436:T1, "Expression out"=w435:T2)  [unwired: 8 in]
            }
            frame "quote" {
              # "return the (1st) argument without any evaluation"
              n189 = Index Array(array=w442, index=0) -> (element=w441:T2)
            }
            frame "while" {
              # "TODO: error checking that all arguments of cond are lists with 2 elements"
              # "(while cond expr)"
              n190 = while {
                tunnel: w445 -> [w453]
                shift-right: [w452] -> w446
                shift-left: w449 -> [w459]
                tunnel: [w451] -> _
                stop <- w450 stop-if-true
                n191 = Index Array(array=w453, index=0) -> (element=w456:T2)
                n192 = call "eval.vi"("Environment in"=w459, "Expression in"=w456) -> ("Environment out"=w455:T1, "Expression out"=w457:T2)  [unwired: 6 in]
                n193 = call "Is True.vi"("Expression in"=w457) -> ("Is True?"=w454:bool)  [unwired: 10 in]
                n194 = case shown="True" w454 {
                  tunnel: w455 -> [w461 w468]
                  tunnel: w453 -> [_ w467]
                  tunnel: [w461 w465] -> w452
                  tunnel: [T2 {"Type"=enum."nil", "Data"=variant} ("Expression out") w464] -> w451
                  tunnel: [TRUE FALSE] -> w450
                  frame False {
                  }
                  frame True {
                    n195 = Index Array(array=w467, index=1) -> (element=w466:T2)
                    n196 = call "eval.vi"("Environment in"=w468, "Expression in"=w466) -> ("Environment out"=w465:T1, "Expression out"=w464:T2)  [unwired: 6 in]
                  }
                }
              }
              n197 = call "eval.vi"("Environment in"=w446) -> ("Environment out"=w448:T1, "Expression out"=w447:T2)  [unwired: 7 in]
            }
            frame Default {
            }
          }
        }
        frame "symbol" {
          n198 = Variant To Data(type="", Variant=w476) -> (data=w473:string)  [unwired: 1 in, 1 out]
          n199 = call "read_environment.vi"("symbol"=w473, "Environment in"=w474) -> ("Expression"=w472:T2)  [unwired: 9 in]
        }
      }
    }
  }
  "Expression out" <- w3
  "Environment out" <- w1
